vi "queryVendorFabricStyle (SubVI).vi"(2 "errorIn":errorcluster, 3 "queryInStr":string, 4 "SampleStyle_0":refnum<vi>, 5 "Mfr_0":refnum<vi>) -> (0 "errorOut":errorcluster, 1 "queryOutStr":string)   [LabVIEW 2015]
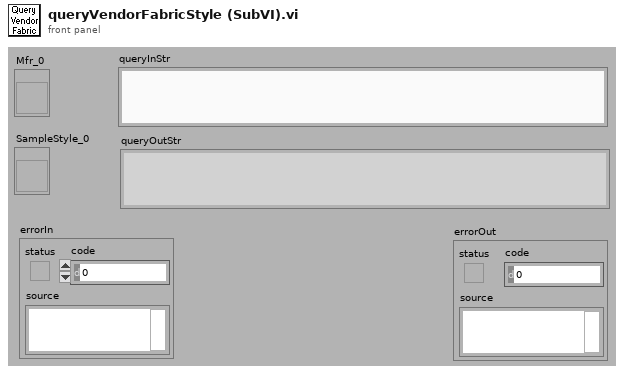
[diagram p1: front panel]
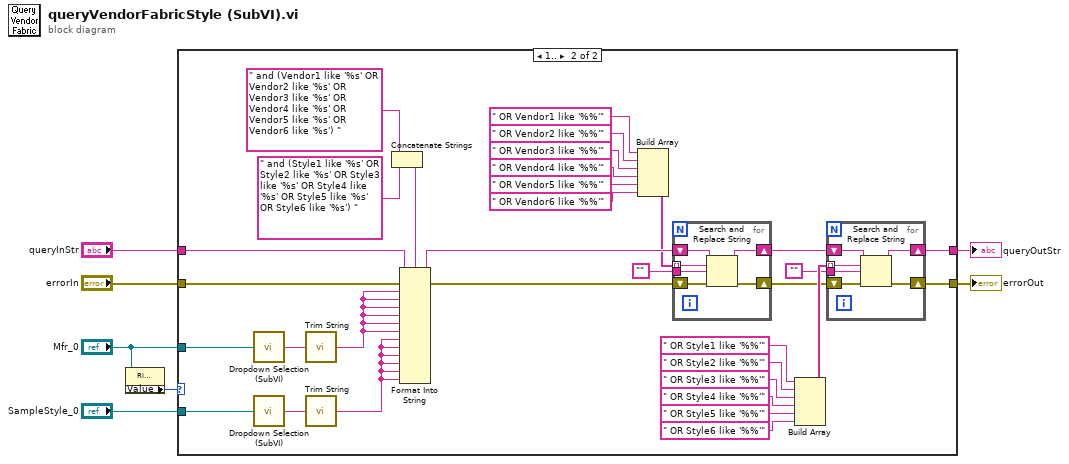
[diagram p0: block diagram]
diagram:
  n1 = property on="Property Node" class="Ring (strict)"(reference="Mfr_0") -> ("Value"=w1:u16)  [unwired: 1 in, 2 out]
  n2 = case shown="1.." w1 {
    tunnel: "Mfr_0" -> [_ w41]
    tunnel: [w9 w14] -> w5
    tunnel: [w8 w13] -> w6
    tunnel: "errorIn" -> [w8 w36]
    tunnel: "queryInStr" -> [w9 w35]
    tunnel: "SampleStyle_0" -> [_ w10]
    frame 0, Default {
    }
    frame 1.. {
      n3 = call "Dropdown Selection (SubVI).vi"("reference"=w41) -> ("element"=w42:string)
      n4 = call "Dropdown Selection (SubVI).vi"("reference"=w10) -> ("element"=w40:string)
      n5 = call "Trim String.vi"("inStr"=w42) -> ("outStr"=w34:string)
      n6 = call "Trim String.vi"("inStr"=w40) -> ("outStr"=w33:string)
      n7 = Concatenate Strings(" and (Vendor1 like '%s' OR Vendor2 like '%s' OR Vendor3 like '%s' OR Vendor4 like '%s' OR Vendor5 like '%s' OR Vendor6 like '%s') " ("Format String"), " and (Style1 like '%s' OR Style2 like '%s' OR Style3 like '%s' OR Style4 like '%s' OR Style5 like '%s' OR Style6 like '%s') " ("Format String")) -> (w39:string)
      n8 = Format Into String(format string=w39, initial string=w35, error in=w36, w34, w34, w34, w34, w34, w34, w33, w33, w33, w33, w33, w33) -> (resulting string=w16:string, error out=w15:errorcluster)
      n9 = Build Array(" OR Vendor1 like '%%'" ("search string"), " OR Vendor2 like '%%'" ("search string"), " OR Vendor3 like '%%'" ("search string"), " OR Vendor4 like '%%'" ("search string"), " OR Vendor5 like '%%'" ("search string"), " OR Vendor6 like '%%'" ("search string")) -> (w12:string[])
      n10 = for {
        shift-right: [w54] -> w23
        shift-left: w16 -> [w53]
        shift-right: [w52] -> w24
        shift-left: w15 -> [w51]
        tunnel: w12 -> [w50] mode=indexing
        tunnel: "" ("replace string (\"\")") -> [w49]
        n11 = Search and Replace String(input string=w53, search string=w50, replace string=w49, error in=w51) -> (result string=w54:string, error out=w52:errorcluster)  [unwired: 6 out]
      }
      n12 = Build Array(" OR Style1 like '%%'" ("search string"), " OR Style2 like '%%'" ("search string"), " OR Style3 like '%%'" ("search string"), " OR Style4 like '%%'" ("search string"), " OR Style5 like '%%'" ("search string"), " OR Style6 like '%%'" ("search string")) -> (w25:string[])
      n13 = for {
        shift-right: [w48] -> w14
        shift-left: w23 -> [w47]
        shift-right: [w46] -> w13
        shift-left: w24 -> [w45]
        tunnel: w25 -> [w44] mode=indexing
        tunnel: "" ("replace string (\"\")") -> [w43]
        n14 = Search and Replace String(input string=w47, search string=w44, replace string=w43, error in=w45) -> (result string=w48:string, error out=w46:errorcluster)  [unwired: 6 out]
      }
    }
  }
  "errorOut" <- w6
  "queryOutStr" <- w5
